vi "Handle REGISTERED.vi"(0 "reference":refnum<class "WAMP Client.lvclass">, 5 "Message Loop Shift Register Data":T1, 7 "WAMP Message":T16 {"Message Codes" items=["HELLO"=1, "WELCOME"=2, "ABORT"=3, "GOODBYE"=6, "ERROR"=8, "PUBLISH"=16, "PUBLISHED"=17, "SUBSCRIBE"=32, "SUBSCRIBED"=33, "UNSUBSCRIBE"=34, "UNSUBSCRIBED"=35, "EVENT"=36, "CALL"=48, "RESULT"=59, "REGISTER"=64, "REGISTERED"=65, "UNREGISTER"=66, "UNREGISTERED"=67, "INVOCATION"=68, "YIELD"=70]}, 11 "error in (no error)":errorcluster) -> (4 "reference out":refnum<class "WAMP Client.lvclass">, 6 "output cluster":T1, 15 "error out":errorcluster)   [LabVIEW 2020, in "wamplv.lvlib" / "WAMP Client.lvclass"]
uses:
  WAMP Client.lvclass
  TypeDef/WAMP Received Message.ctl
  TypeDef/WAMP Message Codes.ctl
  TypeDef/Message Loop Shift Reg Data.ctl
  TypeDef/REGISTER Request Data.ctl
  TypeDef/Success or error.ctl
  API/TypeDefs/Combined error.ctl
  API/TypeDefs/WAMP error.ctl
  API/TypeDefs/INVOCATION payload2.ctl
  TypeDef/Publish Requests Map.ctl
  TypeDef/PUBLISH Request Data.ctl
  TypeDef/PUBLISH result2.ctl
  TypeDef/Endpoint Data.ctl
  TypeDef/CALL Request Map.ctl
  TypeDef/CALL Request Data.ctl
  API/TypeDefs/RESULT payload2.ctl
  TypeDef/SUBSCRIBE Requests Map.ctl
  TypeDef/SUBSCRIBE Request Data.ctl
  TypeDef/Subscribe Result.ctl
  TypeDef/EVENT payload2.ctl
  TypeDef/Subscriptions Map.ctl
  TypeDef/Subscription Details.ctl
  TypeDef/Unsubscribe Requests Map.ctl
  TypeDef/UNSUBSCRIBE Request Data.ctl
  TypeDef/UNSUBSCRIBE Result.ctl
  TypeDef/Unregister requests map.ctl
  TypeDef/Unregister request.ctl
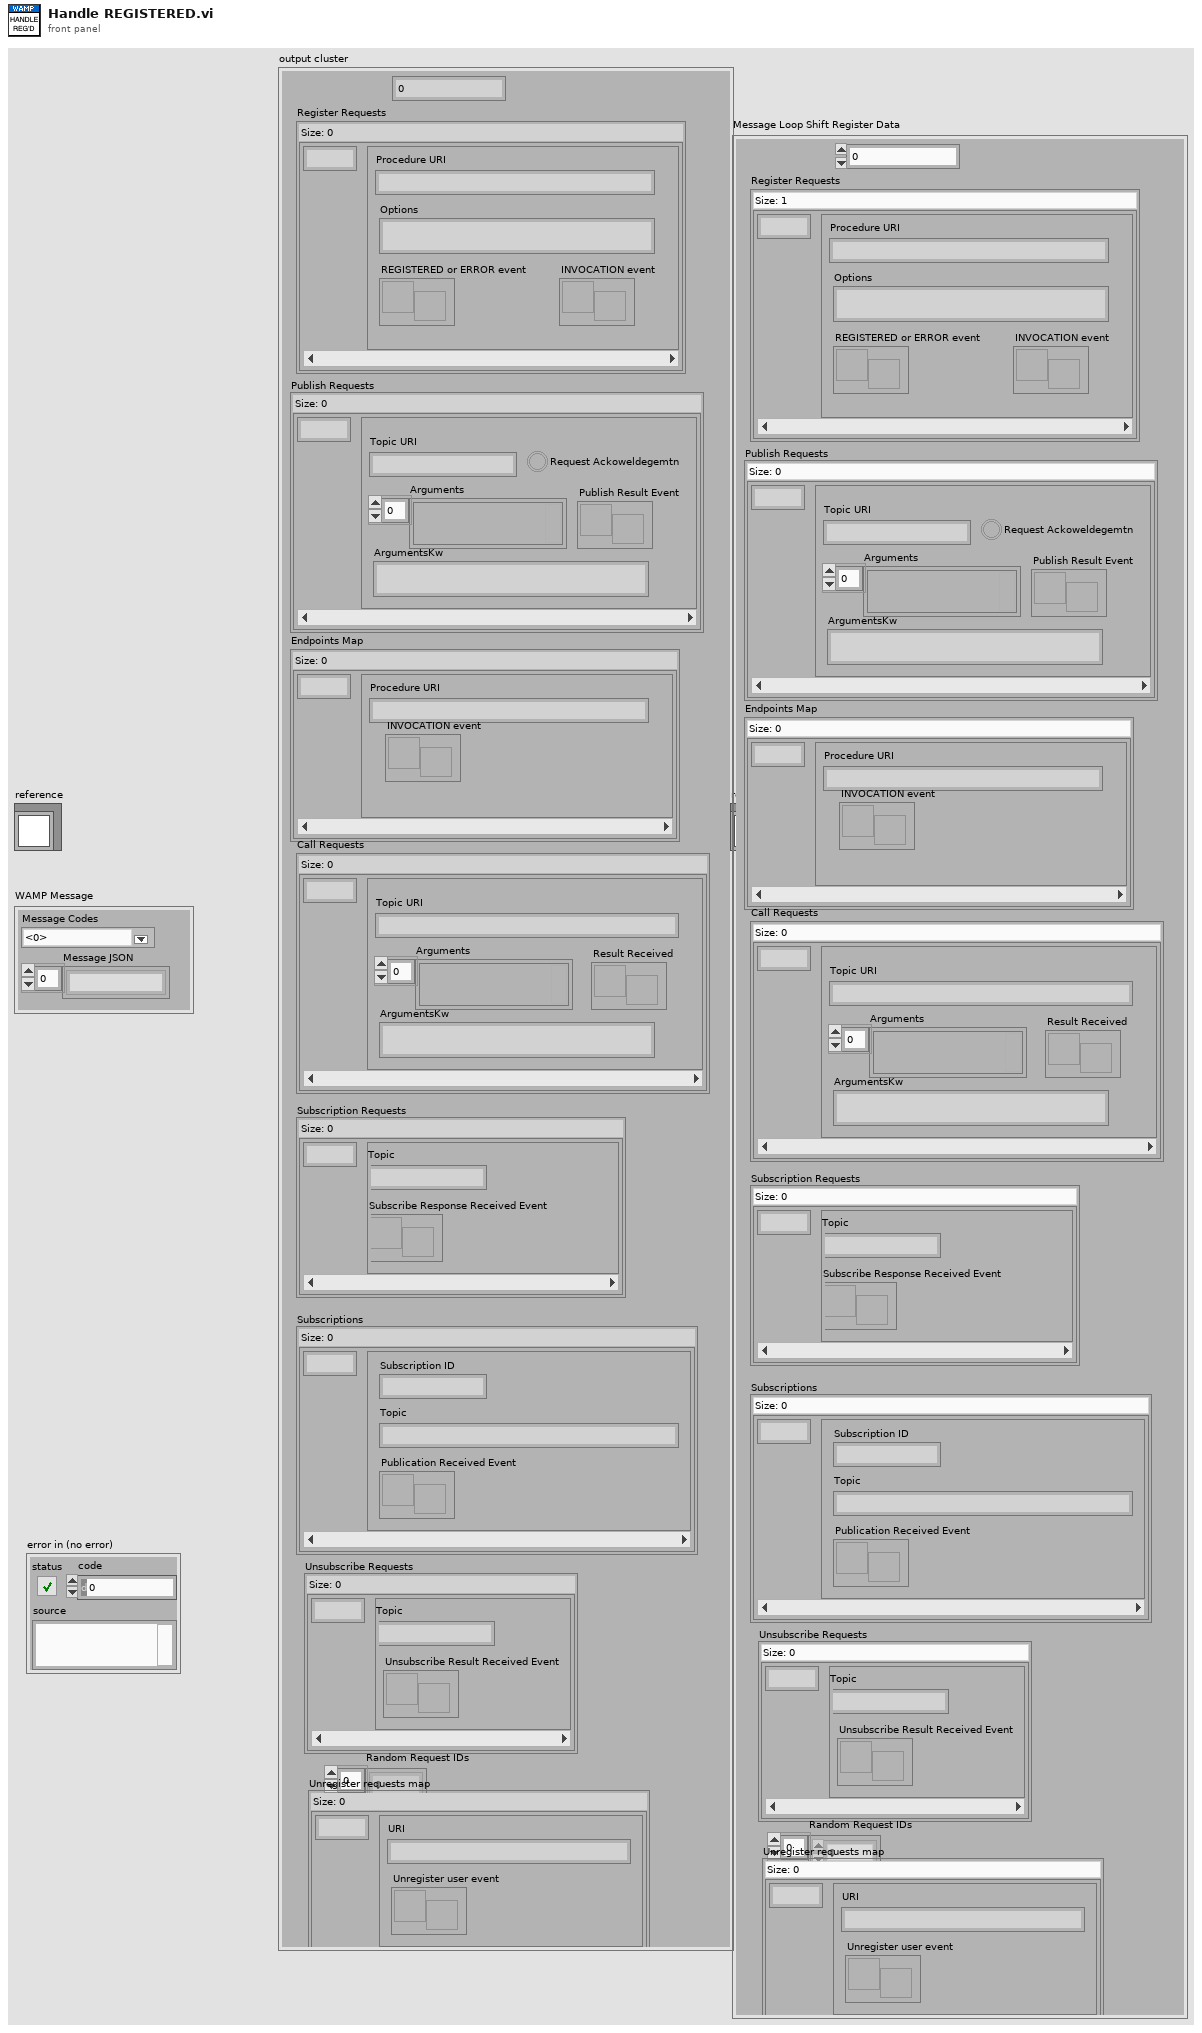
[diagram p1: front panel]
types:
  T1 = typedef "wamplv.lvlib/WAMP Client.lvclass/Message Loop Shift Reg Data.ctl" = cluster{"Last Request ID":u64, "Register Requests":map{u64, T2}, "Publish Requests":T3, "Endpoints Map":map{u64, T5}, "Call Requests":T6, "Subscription Requests":T8, "Subscriptions":T10, "Unsubscribe Requests":T12, "Random Request IDs":u64[], "Unregister requests map":T14}
  T2 = typedef "wamplv.lvlib/WAMP Client.lvclass/REGISTER Request Data.ctl" = cluster{"Procedure URI":string, "Options":string, "REGISTERED or ERROR event":refnum<user-event>, "INVOCATION event":refnum<user-event>}
  T3 = typedef "wamplv.lvlib/WAMP Client.lvclass/Publish Requests Map.ctl" = map{u64, T4}
  T4 = typedef "wamplv.lvlib/WAMP Client.lvclass/PUBLISH Request Data.ctl" = cluster{"Topic URI":string, "Arguments":variant[], "ArgumentsKw":string, "Publish Result Event":refnum<user-event>, "Request Ackoweldegemtn":bool}
  T5 = typedef "wamplv.lvlib/WAMP Client.lvclass/Endpoint Data.ctl" = cluster{"Procedure URI":string, "INVOCATION event":refnum<user-event>}
  T6 = typedef "wamplv.lvlib/WAMP Client.lvclass/CALL Request Map.ctl" = map{u64, T7}
  T7 = typedef "wamplv.lvlib/WAMP Client.lvclass/CALL Request Data.ctl" = cluster{"Topic URI":string, "Arguments":variant[], "ArgumentsKw":string, "Result Received":refnum<user-event>}
  T8 = typedef "wamplv.lvlib/WAMP Client.lvclass/SUBSCRIBE Requests Map.ctl" = map{u64, T9}
  T9 = typedef "wamplv.lvlib/WAMP Client.lvclass/SUBSCRIBE Request Data.ctl" = cluster{"Topic":string, "Subscribe Response Received Event":refnum<user-event>}
  T10 = typedef "wamplv.lvlib/WAMP Client.lvclass/Subscriptions Map.ctl" = map{u64, T11}
  T11 = typedef "wamplv.lvlib/WAMP Client.lvclass/Subscription Details.ctl" = cluster{"Subscription ID":u64, "Topic":string, "Publication Received Event":refnum<user-event>}
  T12 = typedef "wamplv.lvlib/WAMP Client.lvclass/Unsubscribe Requests Map.ctl" = map{u64, T13}
  T13 = typedef "wamplv.lvlib/WAMP Client.lvclass/UNSUBSCRIBE Request Data.ctl" = cluster{"Topic":string, "Unsubscribe Result Received Event":refnum<user-event>}
  T14 = typedef "wamplv.lvlib/WAMP Client.lvclass/Unregister requests map.ctl" = map{u64, T15}
  T15 = typedef "wamplv.lvlib/WAMP Client.lvclass/Unregister request.ctl" = cluster{"URI":string, "Unregister user event":refnum<user-event>}
  T16 = typedef "wamplv.lvlib/WAMP Client.lvclass/WAMP Received Message.ctl" = cluster{"Message JSON":string[], "Message Codes":T17}
  T17 = typedef "wamplv.lvlib/WAMP Client.lvclass/WAMP Message Codes.ctl" = u16
  T18 = typedef "wamplv.lvlib/WAMP Client.lvclass/Success or error.ctl" = cluster{"Success?":bool, "URI":string, "Combined Error":T19}
  T19 = typedef "wamplv.lvlib/WAMP Client.lvclass/Combined error.ctl" = cluster{"Error?":bool, "WAMP Error":T20, "Error":errorcluster}
  T20 = typedef "wamplv.lvlib/WAMP Client.lvclass/WAMP error.ctl" = cluster{"Details":string, "ArgumentKw Payload":string, "Error?":bool, "Error URI":string, "Arguments Payload":string[]}
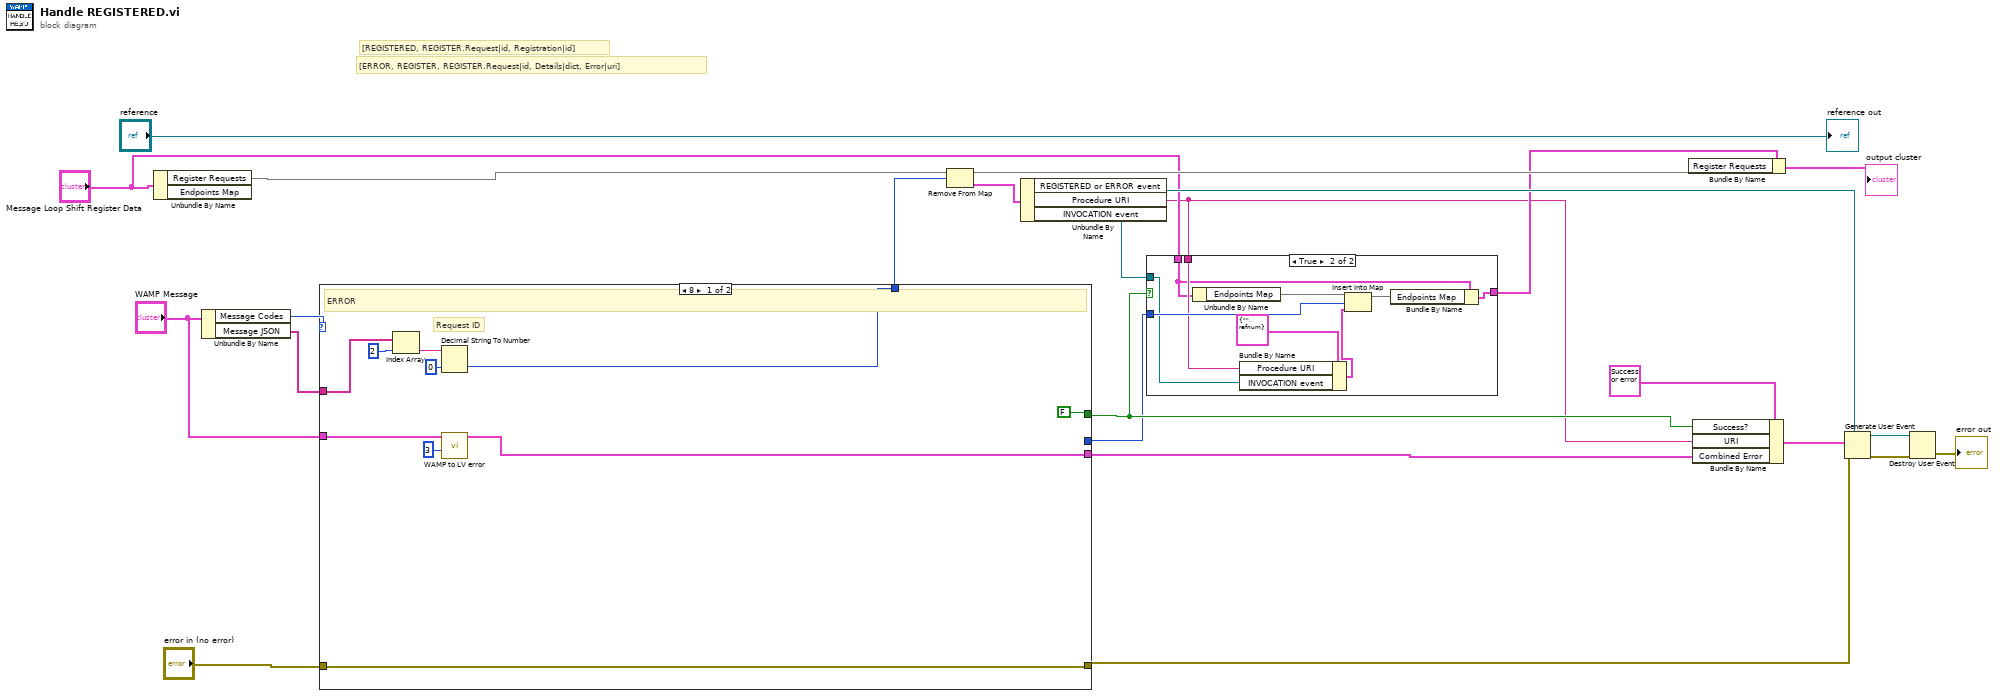
[diagram p0: block diagram]
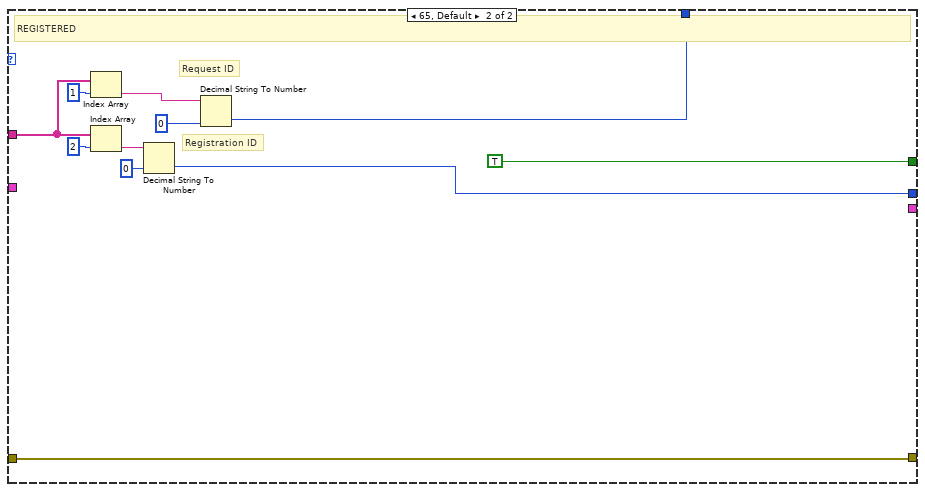
[diagram p3: hidden frame]
diagram:
  # "[ERROR, REGISTER, REGISTER.Request|id, Details|dict, Error|uri]"
  # "[REGISTERED, REGISTER.Request|id, Registration|id]"
  n1 = Unbundle By Name("Message Loop Shift Register Data") -> ("Register Requests"=w14:map{u64, T2})  [unwired: 1 out]
  n2 = Unbundle By Name("WAMP Message") -> ("Message Codes"=w22:T17, "Message JSON"=w21:string[])
  n3 = case shown="8" w22 {
    tunnel: w21 -> [w30 w38]
    tunnel: [w31 w37] -> w12
    tunnel: "error in (no error)" -> [w26 w36]
    tunnel: [w26 w36] -> w23
    tunnel: [FALSE ("Success?") TRUE ("Success?")] -> w8
    tunnel: [_ w35] -> w6
    tunnel: "WAMP Message" -> [w28 _]
    tunnel: [w25 _] -> w1
    frame 8 {
      # "Request ID"
      # "ERROR"
      n4 = Index Array(array=w30, index=u32 2) -> (element=w33:string)
      n5 = Decimal String To Number(string=w33, default (0L)=u32 0) -> (number=w31:u32)  [unwired: 1 in, 1 out]
      n6 = call "WAMP to LV error.vi"("Details Index"=u32 3, "WAMP Message"=w28) -> ("Combined Error"=w25:T19)  [unwired: 7 in, 2 out]
    }
    frame 65, Default {
      # "Request ID"
      # "Registration ID"
      # "REGISTERED"
      n7 = Index Array(array=w38, index=1) -> (element=w41:string)
      n8 = Index Array(array=w38, index=2) -> (element=w44:string)
      n9 = Decimal String To Number(string=w44, default (0L)=u64 0) -> (number=w35:u64)  [unwired: 1 in, 1 out]
      n10 = Decimal String To Number(string=w41, default (0L)=u64 0) -> (number=w37:u64)  [unwired: 1 in, 1 out]
    }
  }
  n11 = Remove From Map(10:w12, 11:w14) -> (1:w20:T2, 3:w10:map{u64, T2})  [unwired: 1 out]
  n12 = Unbundle By Name(w20) -> ("REGISTERED or ERROR event"=w17:refnum<user-event>, "Procedure URI"=w3:string, "INVOCATION event"=w7:refnum<user-event>)
  n13 = case shown="True" w8 {
    tunnel: w7 -> [_ w52]
    tunnel: w6 -> [_ w54]
    tunnel: "Message Loop Shift Register Data" -> [w46 w49]
    tunnel: [w46 w47] -> w4
    tunnel: w3 -> [_ w51]
    frame False {
    }
    frame True {
      n14 = Unbundle By Name(w49) -> ("Endpoints Map"=w55:map{u64, T5})
      n15 = Bundle By Name(cluster=T5 {"Procedure URI"="", "INVOCATION event"=refnum} ("Endpoint Data"), "Procedure URI"=w51, "INVOCATION event"=w52) -> (w50:T5)
      n16 = Insert Into Map(map in=w55, key=w54, value=w50) -> (map out=w48:map{u64, T5})  [unwired: 2 out]
      n17 = Bundle By Name(cluster=w49, "Endpoints Map"=w48) -> (w47:T1)
    }
  }
  n18 = Bundle By Name(cluster=w4, "Register Requests"=w10) -> (→"output cluster":T1)
  n19 = Bundle By Name(cluster=T18 {"Success?"=FALSE, "URI"="", "Combined Error"={"Error?"=FALSE, "WAMP Error"={"Details"="{}", "ArgumentKw Payload"="", "Error?"=FALSE, "Error URI"="", "Arguments Payload"=[]}, "Error"={"status"=FALSE, "code"=0, "source"=""}}} ("REGISTERED or ERROR payload"), "Success?"=w8, "URI"=w3, "Combined Error"=w1) -> (w15:T18)
  n20 = Generate User Event(user event=w17, event data cluster=w15, error in=w23) -> (user event out=w18:refnum<user-event>, error out=w19:errorcluster)  [unwired: 1 in]
  n21 = Destroy User Event(user event=w18, error in=w19) -> (error out=→"error out":errorcluster)
  "reference out" <- "reference"
